vi "Begin.vi"(8 "error in (no error)":errorcluster, 11 "EventMgrFile in":refnum<class "EventMgrFile.lvclass">) -> (0 "error out":errorcluster, 3 "EventMgrFile out":refnum<class "EventMgrFile.lvclass">)   [LabVIEW 2013, in "EventMgrFile.lvclass"]
uses:
  EventMgrFile.lvclass
  EventMgr/EventMgr.lvclass
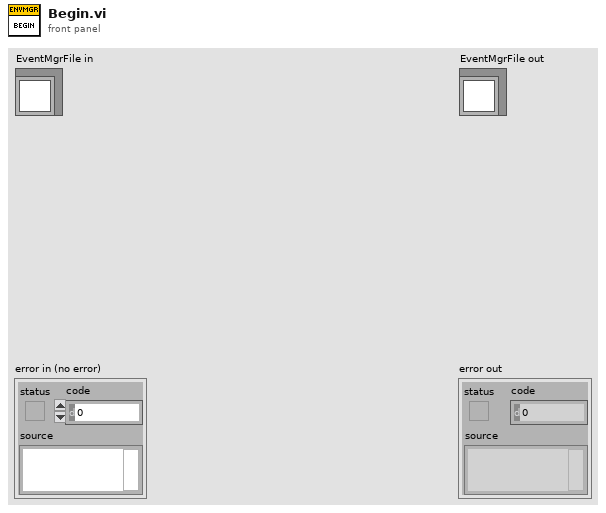
[diagram p1: front panel]
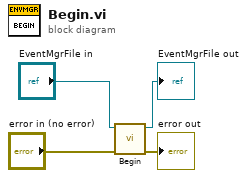
[diagram p0: block diagram]
diagram:
  n1 = call-parent "Begin.vi"("error in (no error)"="error in (no error)", "EventMgr in"="EventMgrFile in") -> ("error out"=→"error out":errorcluster, "EventMgr out"=→"EventMgrFile out":refnum<class "EventMgrFile.lvclass">)  [unwired: 8 in]
